vi "Read Custom Errors.vi"(8 "Error In":errorcluster, 11 "Error.lvclass":refnum<class "Error.lvclass">) -> (0 "Error Out":errorcluster, 2 "Error Codes":i32[](array[numeric]), 3 "Error Messages":string[](array[string]))   [LabVIEW 2019, in "TSC Error.lvlib" / "Error.lvclass"]
doc: "This VI reads the custom error codes form the Error Codes.cfg configuration file. This file has a list of defined errors specified by the project.\n\nInputs:\n-error in (no error)\n\nOutputs:\n-Error Messages [array of strings] - the custom error messages\n-Error Codes [array of I32's] - the custom error codes\n-error out\n________________________________________________________________________________\n<b>Code Developed By:</b>\nDaniel Coons\nTechnology Service Corporation\n1983 S Liberty Drive\nBloomington, IN 47403\nPhone: 812 558-7100\ndaniel.coons@tsc.com\nwww.tsc.com\n\n<b>Date Created:</b> 12 AUG 2014\n<b>Date Updated:</b>"
uses:
  Error.lvclass
  Error.lvclass/Error.ctl
  <vilib>/Utility/config.llb/Read Key (String).vi
  <vilib>/Utility/config.llb/NI_LVConfig.lvlib
  TSC Error.lvlib
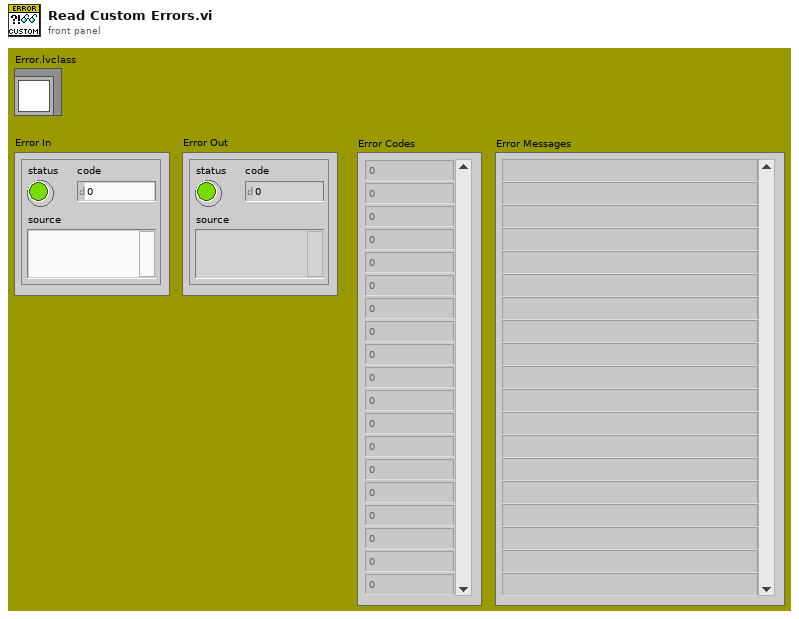
[diagram p1: front panel]
types:
  T1 = typedef "NI_LVConfig.lvlib/Config Data RefNum.ctl" = refnum<k1>
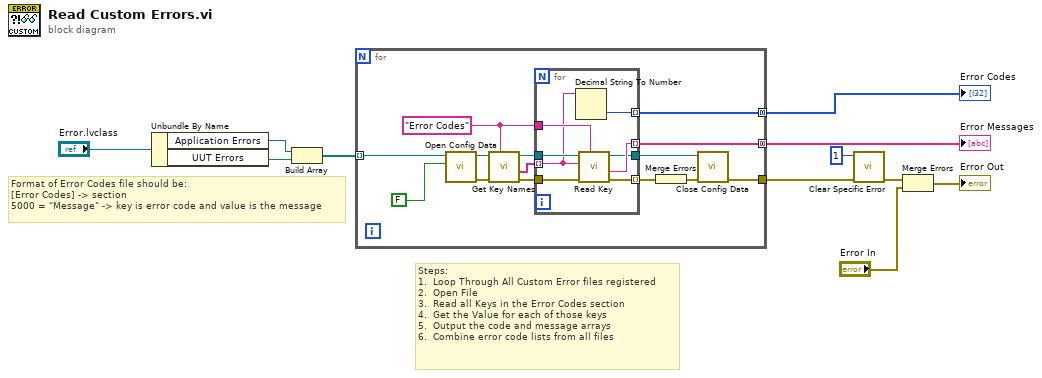
[diagram p0: block diagram]
diagram:
  # "Format of Error Codes file should be:\n[Error Codes] -> section\n5000 = \"Message\" -> key is error code and value is the message"
  # "Steps:\n1.  Loop Through All Custom Error files registered\n2.  Open File\n3.  Read all Keys in the Error Codes section\n4.  Get the Value for each of those keys\n5.  Output the code and message arrays\n6.  Combine error code lists from all files"
  n1 = Unbundle By Name("Error.lvclass") -> ("Application Errors"=w2:path, "UUT Errors"=w3:path)
  n2 = Build Array(w2, w3) -> (w1:path[])
  n3 = for {
    tunnel: [w25] -> w10 mode=concatenating
    tunnel: [w24] -> w9 mode=concatenating
    tunnel: [w13] -> w5
    tunnel: w1 -> [w12] mode=indexing
    w17 = "Error Codes" ("section")
    n4 = call <vilib>:"Open Config Data.vi"("create file if necessary (T)"=FALSE, "configuration file path"=w12) -> ("error out"=w22:errorcluster, "refnum"=w21:T1)  [unwired: 7 in, 1 out]
    n5 = call <vilib>:"Get Key Names.vi"("section"=w17, "error in (no error)"=w22, "refnum"=w21) -> ("error out"=w19:errorcluster, "key names"=w18:string[], "refnum out"=w20:T1)  [unwired: 5 in, 1 out]
    n6 = for {
      tunnel: w20 -> [w33]
      tunnel: w19 -> [w32]
      tunnel: w18 -> [w27] mode=indexing
      tunnel: w17 -> [w31]
      tunnel: [w30] -> w25 mode=indexing
      tunnel: [w29] -> w16
      tunnel: [w28] -> w15 mode=indexing
      tunnel: [w26] -> w24 mode=indexing
      n7 = Decimal String To Number(string=w27) -> (number=w26:i32)  [unwired: 2 in, 1 out]
      n8 = call-poly <vilib>:"Read Key.vi"("section"=w31, "error in (no error)"=w32, "key"=w27, "refnum"=w33) -> ("error out"=w28:errorcluster, "value"=w30:string, "refnum out"=w29:T1)  [unwired: 4 in, 1 out]
    }
    n9 = Merge Errors(w15) -> (w14:errorcluster)
    n10 = call <vilib>:"Close Config Data.vi"("error in (no error)"=w14, "refnum"=w16) -> ("error out"=w13:errorcluster)  [unwired: 8 in, 1 out]
  }
  "Error Messages" <- w10
  "Error Codes" <- w9
  n11 = call "Clear Specific Error.vi"("error in"=w5, "Error Code"=1 ("ErrorCodeToClear")) -> ("error out"=w7:errorcluster)  [unwired: 9 in]
  n12 = Merge Errors(w7, "Error In") -> (→"Error Out":errorcluster)
